vi "WriteDataTDMS.vi"(4 "SignalOut":waveform(dbl), 5 "Accel.":waveform(dbl), 7 "TDMS Input":refnum<k34>, 9 "Identifier":enum16{"Accel", "SignalOut", "ButtonPress"}(ring), 11 "InputDataType":enum16{"Waveform", "DBL"}(ring)=enum."DBL", 13 "TimeInterval":i64, 15 "ActualStart[f]":i64, 17 "Accel":dbl[](array[numeric]), 19 "SignalOut":dbl[](array[numeric])) -> (0 "tdms file out":refnum<k34>, 18 "error out":errorcluster)   [LabVIEW 2022 SP3]
uses:
  <vilib>/Utility/error.llb/DialogType.ctl
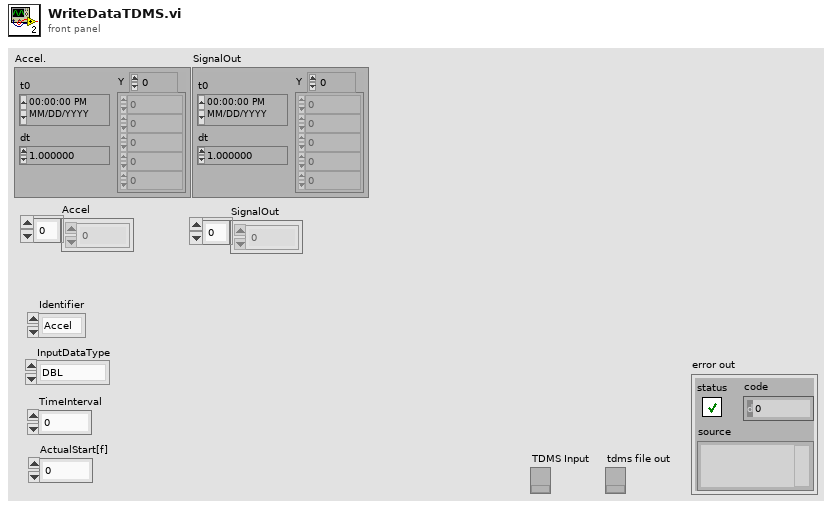
[diagram p1: front panel]
types:
  T1 = typedef "DialogType.ctl" = u16
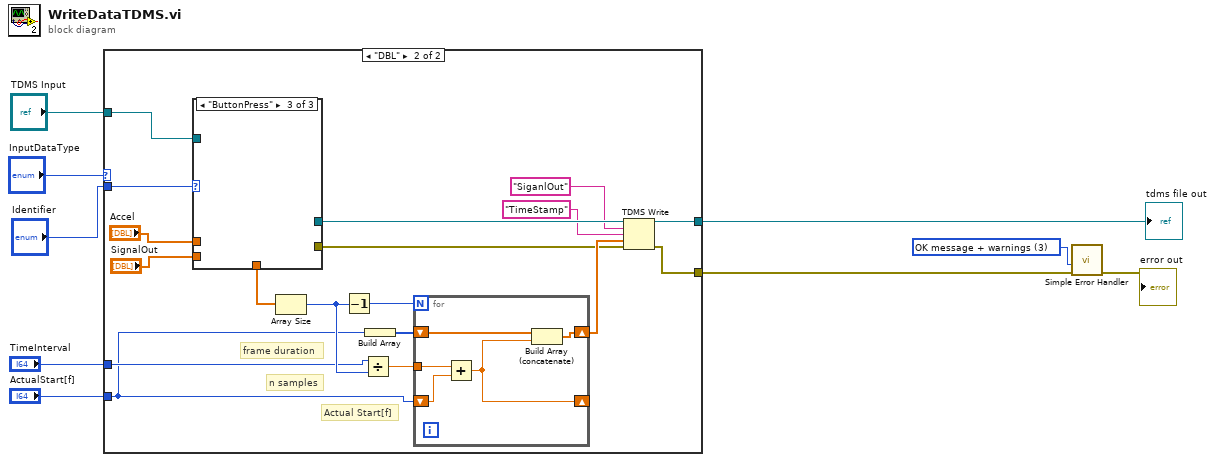
[diagram p0: block diagram]
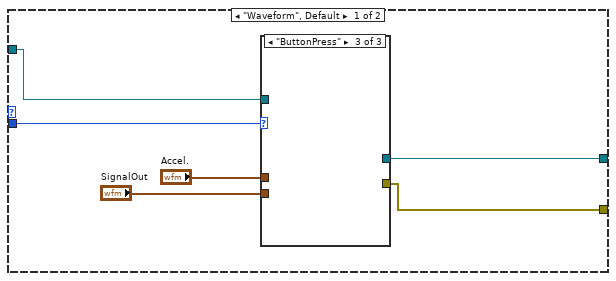
[diagram p2: hidden frame]
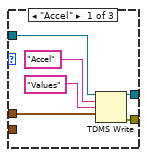
[diagram p3: hidden frame]
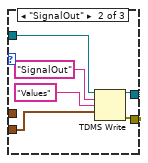
[diagram p4: hidden frame]
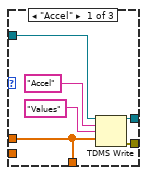
[diagram p5: hidden frame]
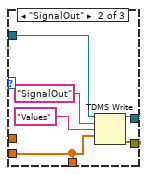
[diagram p6: hidden frame]
diagram:
  w9 = T1 3 items=["no dialog", "OK message", "continue or stop message", "OK message + warnings", "continue/stop + warnings"] ("type of dialog (OK msg:1)")
  n1 = case shown="\"DBL\"" "InputDataType" {
    tunnel: "TDMS Input" -> [w12 w38]
    tunnel: "Identifier" -> [w13 w37]
    tunnel: "ActualStart[f]" -> [_ w35]
    tunnel: "TimeInterval" -> [_ w36]
    tunnel: [w10 w29] -> w2
    tunnel: [w11 w28] -> w1
    frame "Waveform", Default {
      n2 = case shown="\"ButtonPress\"" w13 {
        tunnel: [w19 w25 _] -> w10
        tunnel: [w18 w24 _] -> w11
        tunnel: "Accel." -> [w17 _ _]
        tunnel: "SignalOut" -> [_ w23 _]
        tunnel: w12 -> [w16 w22 _]
        frame "Accel" {
          n3 = TDMS Write(0:w16, 5:"Accel" ("group name in (Untitled)"), 7:"Values", 9:w17) -> (4:w18:refnum<k34>, 15:w19:errorcluster)  [unwired: 2 in, 2 out]
        }
        frame "SignalOut" {
          n4 = TDMS Write(0:w22, 5:"SignalOut" ("group name in (Untitled)"), 7:"Values", 9:w23) -> (4:w24:refnum<k34>, 15:w25:errorcluster)  [unwired: 2 in, 2 out]
        }
        frame "ButtonPress" {
        }
      }
    }
    frame "DBL" {
      # "Actual Start[f]"
      # "n samples"
      # "frame duration"
      n5 = case shown="\"ButtonPress\"" w37 {
        tunnel: [w54 w60 _] -> w30
        tunnel: [w53 w59 _] -> w34
        tunnel: "Accel" -> [w52 _ _]
        tunnel: "SignalOut" -> [_ w58 _]
        tunnel: [w52 w58 _] -> w39
        tunnel: w38 -> [w51 w57 _]
        frame "Accel" {
          n6 = TDMS Write(0:w51, 5:"Accel" ("group name in (Untitled)"), 7:"Values", 9:w52) -> (4:w53:refnum<k34>, 15:w54:errorcluster)  [unwired: 2 in, 2 out]
        }
        frame "SignalOut" {
          n7 = TDMS Write(0:w57, 5:"SignalOut" ("group name in (Untitled)"), 7:"Values", 9:w58) -> (4:w59:refnum<k34>, 15:w60:errorcluster)  [unwired: 2 in, 2 out]
        }
        frame "ButtonPress" {
        }
      }
      n8 = Array Size(array=w39) -> (size(s)=w40:i32)
      n9 = Decrement(x=w40) -> (x-1=w41:i32)
      n10 = Divide(x=w36, y=w40) -> (x/y=w43:dbl)
      n11 = Build Array(w35) -> (w42:i64[])
      n12 = for {
        N: w41 -> [_]
        shift-right: [w47] -> _
        shift-left: w35 -> [w50]
        shift-right: [w49] -> w31
        shift-left: w42 -> [w48]
        tunnel: w43 -> [w46]
        n13 = Add(x=w46, y=w50) -> (x+y=w47:dbl)
        n14 = Build Array (concatenate)(w48, w47) -> (w49:dbl[])
      }
      n15 = TDMS Write(0:w34, 5:"SiganlOut" ("group name in (Untitled)"), 7:"TimeStamp", 9:w31, 11:w30) -> (4:w28:refnum<k34>, 15:w29:errorcluster)  [unwired: 1 in, 2 out]
    }
  }
  "tdms file out" <- w1
  n16 = call <vilib>:"Simple Error Handler.vi"("type of dialog (OK msg:1)"=w9, "error in (no error)"=w2) -> ("error out"=→"error out":errorcluster)  [unwired: 3 in, 4 out]
